vi "TestInsertIntoPanel_OK.vi"(8 "error in (no error)":errorcluster, 11 "TestCase in":refnum<class "TestProtectedSubpanel.lvclass">) -> (0 "error out":errorcluster, 3 "TestCase out":refnum<class "TestProtectedSubpanel.lvclass">)   [LabVIEW 2017, in "TestProtectedSubpanel.lvclass"]
uses:
  TestProtectedSubpanel.lvclass
  TestProtectedSubpanel.lvclass/TestProtectedSubpanel.ctl
  Doubles/ViewableOne/ViewableOne.lvclass
  Source/IViewable/IViewable/IViewable.lvclass/IViewable.ctl
  Source/IViewable/ProtectedSubpanel/ProtectedSubpanel.lvclass/ProtectedSubpanel.ctl
  Source/IViewable/ProtectedSubpanel/Evaluate Insertion Request.vi
  Source/IViewable/IViewable/Evaluate Destination Subpanel.vi
  Source/IViewable/ProtectedSubpanel/Do Insertion.vi
  Source/IViewable/IViewable/IViewable.lvclass
  Source/IViewable/ProtectedSubpanel/ProtectedSubpanel.lvclass
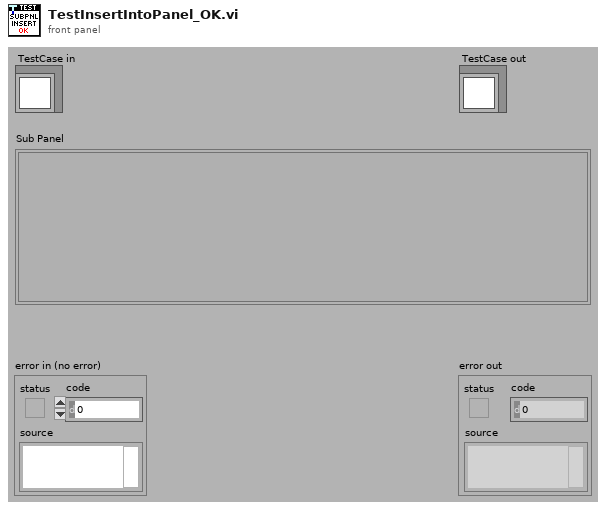
[diagram p1: front panel]
types:
  T1 = typedef "IViewable.lvlib/ProtectedSubpanel.lvclass/Protected Subpanel Reference.ctl" = refnum<data-value>
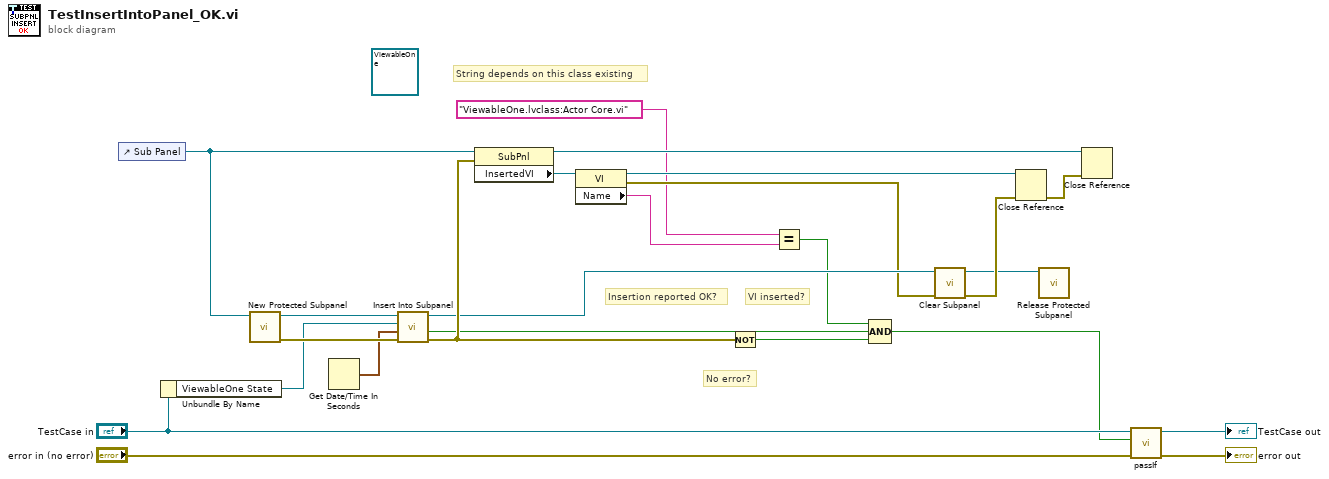
[diagram p0: block diagram]
diagram:
  (unwired) refnum<class "ViewableOne.lvclass"> refnum ("ViewableOne.lvclass")
  # "String depends on this class existing"
  # "Insertion reported OK?"
  # "No error?"
  # "VI inserted?"
  n1 = control-ref of="Sub Panel"() -> (w1:refnum<vi>)
  n2 = Unbundle By Name("TestCase in") -> ("ViewableOne State"=w6:refnum<class "IViewable.lvclass">)
  n3 = call "New Protected Subpanel.vi"("SubPnl Refnum"=w1) -> ("error out"=w13:errorcluster, "Protected Subpanel"=w21:T1)  [unwired: 9 in]
  n4 = Get Date/Time In Seconds() -> (seconds since 1Jan1904=w12:timestamp)
  n5 = call "Insert Into Subpanel.vi"("error in (no error)"=w13, "Insertion Request Time"=w12, "Viewable"=w6, "Protected Subpanel"=w21) -> ("error out"=w19:errorcluster, "Inserted?"=w11:bool, "Protected Subpanel"=w14:T1)  [unwired: 4 in, 1 out]
  n6 = property class="SubPnl"(reference=w1, error in=w19) -> (reference out=w16:refnum<vi>, "InsertedVI"=w18:refnum<vi>)  [unwired: 1 out]
  n7 = property class="VI"(reference=w18) -> (reference out=w8:refnum<vi>, error out=w5:errorcluster, "Name"=w17:string)  [unwired: 1 in]
  n8 = Not(x=w19) -> (.not. x?=w20:bool)
  n9 = Equal?(x="ViewableOne.lvclass:Actor Core.vi" ("y"), y=w17) -> (x = y?=w9:bool)
  n10 = Compound Arithmetic op=AND(w9, w11, w20) -> (w4:bool)
  n11 = call "Clear Subpanel.vi"("error in (no error)"=w5, "Protected Subpanel"=w14) -> ("error out"=w7:errorcluster, "Protected Subpanel Out"=w2:T1)  [unwired: 8 in]
  n12 = Close Reference(reference=w8, error in (no error)=w7) -> (error out=w15:errorcluster)
  n13 = call "Release Protected Subpanel.vi"("Protected Subpanel"=w2) -> ()  [unwired: 10 in, 1 out]
  n14 = Close Reference(reference=w16, error in (no error)=w15) -> ()  [unwired: 1 out]
  n15 = call-dynamic "passIf.vi"("error in (no error)"="error in (no error)", "pass"=w4, "TestCase in"="TestCase in") -> ("error out"=→"error out":errorcluster, "TestCase out"=→"TestCase out":refnum<class "TestProtectedSubpanel.lvclass">)  [unwired: 7 in]
